vi "Parse Engine Data.vi"(11 "Input":string) -> (1 "Temperature":string, 3 "RPMs":string)   [LabVIEW 2017]
uses:
  <vilib>/regexp/Match Regular Expression.xnode
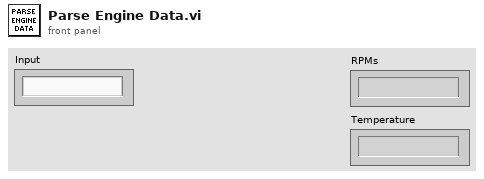
[diagram p1: front panel]
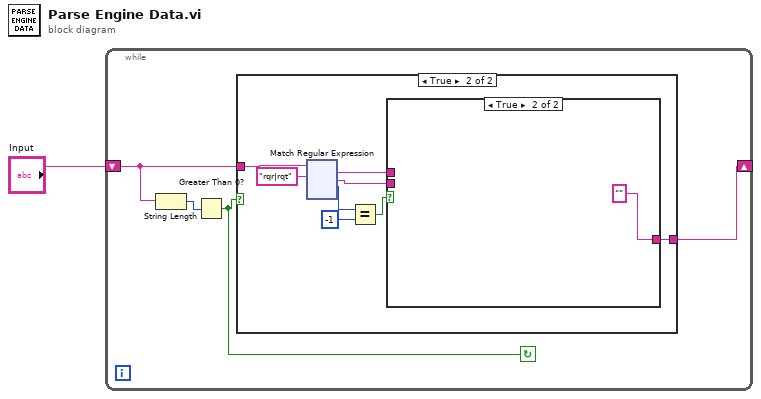
[diagram p0: block diagram]
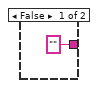
[diagram p2: hidden frame]
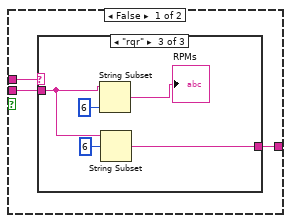
[diagram p3: hidden frame]
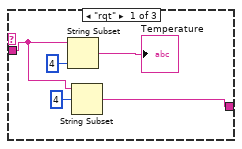
[diagram p4: hidden frame]
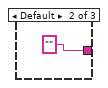
[diagram p5: hidden frame]
diagram:
  n1 = while {
    shift-right: [w2] -> _
    shift-left: "Input" -> [w5]
    stop <- w3 continue-if-true
    n2 = String Length(string=w5) -> (length=w4:i32)
    n3 = Greater Than 0?(x=w4) -> (x > 0?=w3:bool)
    n4 = case shown="True" w3 {
      tunnel: w5 -> [_ w11]
      tunnel: ["" ("after match") w7] -> w2
      frame False {
      }
      frame True {
        n5 = xnode "Match Regular Expression"("input string"=w11, "regular expression"="rqr|rqt") -> ("whole match"=w13:string, "after match"=w12:string, "offset past match"=w10:i32)  [unwired: 4 in, 2 out]
        n6 = Equal?(x=w10, y=-1) -> (x = y?=w8:bool)
        n7 = case shown="True" w8 {
          tunnel: w13 -> [w17 _]
          tunnel: w12 -> [w16 _]
          tunnel: [w15 ""] -> w7
          frame False {
            n8 = case shown="\"rqr\"" w17 {
              tunnel: w16 -> [w19 _ w26]
              tunnel: [w18 "" w24] -> w15
              frame "rqt" {
                n9 = String Subset(string=w19, length (rest)=4 ("length (rest)")) -> (substring=→"Temperature":string)  [unwired: 1 in]
                n10 = String Subset(string=w19, offset (0)=4) -> (substring=w18:string)  [unwired: 1 in]
              }
              frame Default {
              }
              frame "rqr" {
                n11 = String Subset(string=w26, length (rest)=6 ("length (rest)")) -> (substring=→"RPMs":string)  [unwired: 1 in]
                n12 = String Subset(string=w26, offset (0)=6) -> (substring=w24:string)  [unwired: 1 in]
              }
            }
          }
          frame True {
          }
        }
      }
    }
  }
